vi "User_Database_Open.vi"(8 "error in (no error)":errorcluster caption="错误输入（无错误）", 11 "db Path":path=path "00_Database.db") -> (0 "error out":errorcluster caption="错误输出", 3 "SQLite Connection":refnum<class "Connection.lvclass">)   [LabVIEW 2020]
uses:
  <vilib>/drjdpowell/SQLite Library/SQL Connection/Connection.lvclass
  <vilib>/drjdpowell/SQLite Library/SQL Connection/Open (path).vi
  <vilib>/drjdpowell/SQLite Library/SQL Connection/Open (string).vi
  <vilib>/AdvancedString/Path To Command Line String.vi
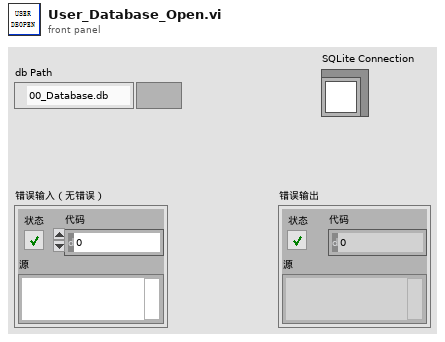
[diagram p1: front panel]
types:
  T1 = enum16{"New or existing", "Existing", "Read only"}
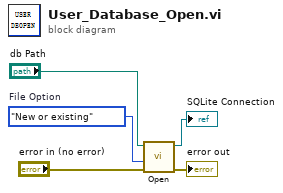
[diagram p0: block diagram]
diagram:
  w4 = T1."New or existing"  # File Option
  n1 = call-poly <vilib>:"Open.vi"("error in (no error)"="error in (no error)", "File Option"=w4, "db file"="db Path") -> ("error out"=→"error out":errorcluster, "SQLite Connection"=→"SQLite Connection":refnum<class "Connection.lvclass">)  [unwired: 7 in]
